vi "PwF_Venom_Open.vi"(8 "error in":errorcluster, 9 "Invert":bool, 10 "Device Number":u8) -> (0 "error out":errorcluster, 3 "Venom Ref":T1={"DeviceStatus"={"status"=FALSE, "code"=0, "source"=""}, "Type"=enum."PWM", "PWM"={"PWM Channel"=enum."PWM 1", "DeadBand"={"Name"="", "maxPositivePwm"=0, "minPositivePwm"=0, "centerPwm"=0, "maxNegativePwm"=0, "minNegativePwm"=0, "angularRange"=0}}, "CAN"={"Device Number"=0, "SetOutput VI Ref"=variant(enum8{"Percent VBus", "Current", "Speed", "Position", "Voltage"} enum."Percent VBus"), "GetOutput VI Ref"=variant(refnum<k1> refnum), "Enable VI Ref"=variant(dbl 12.0), "Disable VI Ref"=variant(enum8{"Percent VBus", "Speed", "Position", "Slave", "Unchanged / Invalid", "Voltage Compensation", "Current", "Motion Profile"} enum."Percent VBus"), "Data"=variant}, "Invert"=FALSE, "DIO PWM"={"PWM \"Enable\" Channel"=enum."Invalid", "DIOChannel"=enum."Invalid", "PWM Rate"=0.0}})   [LabVIEW 2018, in "PwF_Venom.lvlib"]
uses:
  PwF_Venom.lvlib
  <vilib>/Rock Robotics/WPI/MotorControl/WPI_MotorControlDeviceRef.ctl
  <vilib>/Rock Robotics/WPI/MotorControl/WPI_MotorControlType.ctl
  <vilib>/Rock Robotics/SystemInterfaces/DIO/FPGA_DIOPWMChannel.ctl
  <vilib>/Rock Robotics/WPI/PWM/WPI_PWMDeadband.ctl
  <vilib>/Rock Robotics/SystemInterfaces/DIO/FPGA_DIOChannel.ctl
  TypeDefs/PwF_Venom_DevRefData.ctl
  TypeDefs/PwF_Venom_ControlMode.ctl
  <vilib>/Rock Robotics/WPI/ThirdParty/Phoenix-LabVIEW/Controls/DriverLib.ctl
  <vilib>/Rock Robotics/SystemInterfaces/NetworkCommunication/NetComm_UsageReport_ResourceType.ctl
  PwF_Venom_WPISet.vi
  PwF_Venom_Disable.vi
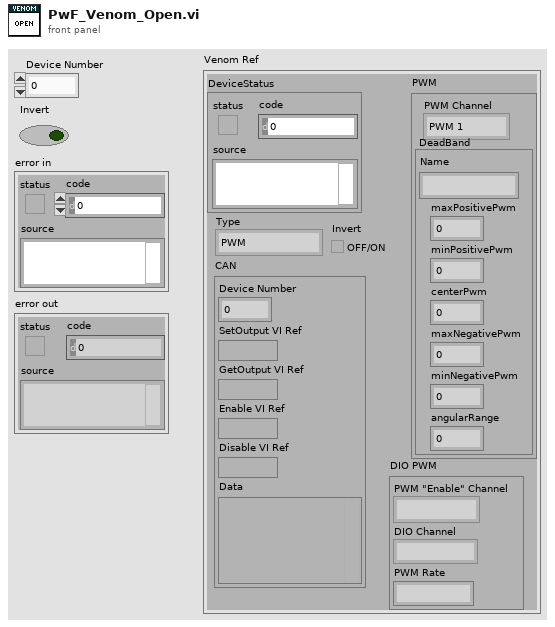
[diagram p1: front panel]
types:
  T1 = typedef "WPI_MotorControlDeviceRef.ctl" = cluster{"DeviceStatus":errorcluster, "Type":T2, "PWM":cluster{"PWM Channel":T3, "DeadBand":T4}, "CAN":cluster{"Device Number":u8, "SetOutput VI Ref":variant, "GetOutput VI Ref":variant, "Enable VI Ref":variant, "Disable VI Ref":variant, "Data":variant}, "Invert":bool, "DIO PWM":cluster{"PWM \"Enable\" Channel":T3, "DIOChannel":T5, "PWM Rate":dbl}}
  T2 = typedef "WPI_MotorControlType.ctl" = enum16{"PWM", "CAN", "DIO PWM"}
  T3 = typedef "FPGA_DIOPWMChannel.ctl" = enum8{"PWM 0", "PWM 1", "PWM 2", "PWM 3", "PWM 4", "PWM 5", "PWM 6", "PWM 7", "PWM 8", "PWM 9", "PWM MXP 0", "PWM MXP 1", "PWM MXP 2", "PWM MXP 3", "PWM MXP 4", "PWM MXP 5", "PWM MXP 6", "PWM MXP 7", "PWM MXP 8", "PWM MXP 9", "Invalid"}
  T4 = typedef "WPI_PWMDeadband.ctl" = cluster{"Name":string, "maxPositivePwm":i32, "minPositivePwm":i32, "centerPwm":i32, "maxNegativePwm":i32, "minNegativePwm":i32, "angularRange":u16}
  T5 = typedef "FPGA_DIOChannel.ctl" = enum8{"DIO 0", "DIO 1", "DIO 2", "DIO 3", "DIO 4", "DIO 5", "DIO 6", "DIO 7", "DIO 8", "DIO 9", "DIO MXP 0", "DIO MXP 1", "DIO MXP 2", "DIO MXP 3", "DIO MXP 4", "DIO MXP 5", "DIO MXP 6", "DIO MXP 7", "DIO MXP 8", "DIO MXP 9", "DIO MXP 10", "DIO MXP 11", "DIO MXP 12", "DIO MXP 13", "DIO MXP 14", "DIO MXP 15", "SPI Port CS1", "SPI Port CS2", "SPI Port CS3", "SPI Port MISO", "SPI Port MOSI", "Invalid"}
  T6 = typedef "PwF_Venom.lvlib/PwF_Venom_DevRefData.ctl" = cluster{"Library":path, "Handle":u64, "Control Mode":T7, "RefNum Name":string}
  T7 = typedef "PwF_Venom.lvlib/PwF_Venom_ControlMode.ctl" = u8
  T8 = typedef "NetComm_UsageReport_ResourceType.ctl" = enum8{"Controller", "Module", "Language", "CANPlugin", "Accelerometer", "ADXL345", "AnalogChannel", "AnalogTrigger", "AnalogTriggerOutput", "CANJaguar", "Compressor", "Counter", "Dashboard", "DigitalInput", "DigitalOutput", "DriverStationCIO", "DriverStationEIO", "DriverStationLCD", "Encoder", "GearTooth", "Gyro", "I2C", "Framework", "Jaguar", "Joystick", "Kinect", "KinectStick", "PIDController", "Preferences", "PWM", "Relay", "RobotDrive", "SerialPort", "Servo", "Solenoid", "SPI", "Task", "Ultrasonic", "Victor", "Button", "Command", "AxisCamera", "PCVideoServer", "SmartDashboard", "Talon", "HiTechnicColorSensor", "HiTechnicAccel", "HiTechnicCompass", "SRF08", "AnalogOutput", "Victor SP", "Talon SRX", "CAN Talon SRX", "ADXL362 Accel", "ADXRS450 Gyro", "Rev SPARK", "Mindsensors SD540", "Digital Filter", "ADIS16448", "PDP", "PCM", "PigeonIMU", "Nidec Brushless", "CTRE CANifier", "CTRE Future 0", "CTRE Future 1", "CTRE Future 2", "CTRE Future 3", "CTRE Future 4", "CTRE Future 5", "CTRE Future 6", "Linear Filter", "Xbox Controller", "USB Camera", "NavX", "Pixy", "Pixy2", "ScanseSweep", "Shuffleboard", "CAN", "Digilent DMC60", "PWM Victor SPX", "Rev SPARK MAX PWM", "Rev SPARK MAX CAN", "ADIS16470"}
  T9 = typedef "DriverLib.ctl" = path
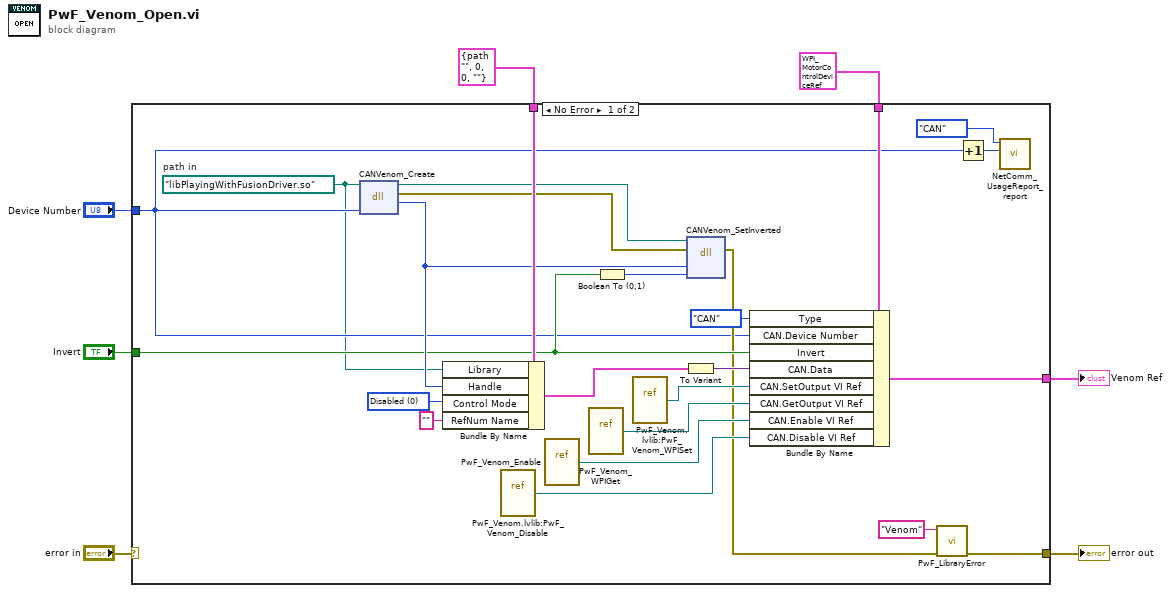
[diagram p0: block diagram]
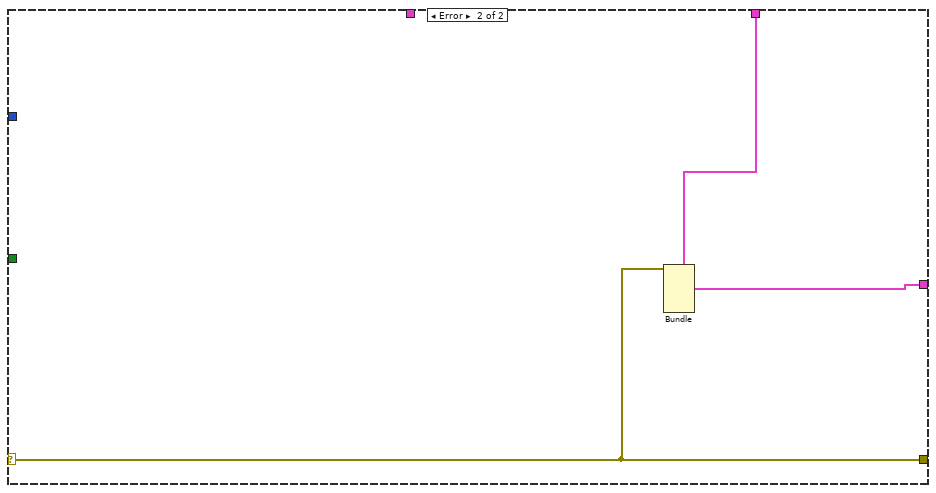
[diagram p2: hidden frame]
diagram:
  n1 = case shown="No Error" "error in" {
    selector: "error in" -> [_ w32]
    tunnel: [w17 w32] -> w7
    tunnel: "Invert" -> [w20 _]
    tunnel: T1 {"DeviceStatus"={"status"=FALSE, "code"=0, "source"=""}, "Type"=enum."CAN", "PWM"={"PWM Channel"=enum."PWM 1", "DeadBand"={"Name"="", "maxPositivePwm"=0, "minPositivePwm"=0, "centerPwm"=0, "maxNegativePwm"=0, "minNegativePwm"=0, "angularRange"=0}}, "CAN"={"Device Number"=0, "SetOutput VI Ref"=variant(refnum<vi> refnum), "GetOutput VI Ref"=variant(refnum<vi> refnum), "Enable VI Ref"=variant(refnum<vi> refnum), "Disable VI Ref"=variant(refnum<vi> refnum), "Data"=variant(cluster{"Control Mode":enum8{"Percent VBus", "Speed", "Position", "Slave", "Unchanged / Invalid", "Voltage Compensation", "Current", "Motion Profile"}, "Encoder Initial Position":dbl, "MaxVout":dbl} {"Control Mode"=enum."Percent VBus", "Encoder Initial Position"=0.0, "MaxVout"=12.0})}, "Invert"=FALSE, "DIO PWM"={"PWM \"Enable\" Channel"=enum."Invalid", "DIOChannel"=enum."Invalid", "PWM Rate"=0.0}} ("CAN Talon SRX Ref") -> [w31 w34]
    tunnel: "Device Number" -> [w12 _]
    tunnel: [w8 w33] -> w1
    tunnel: T6 {"Library"=path "", "Handle"=0, "Control Mode"=0, "RefNum Name"=""} -> [w23 _]
    frame No Error {
      w10 = T7 0 items=["Disabled"=0, "Proportional"=1, "Current Control"=3, "Speed Control"=4, "Position Control"=5, "Motion Profile"=6, "Follow The Leader"=7, "Voltage Control"=8] ("Control Mode")
      w9 = T9 path "libPlayingWithFusionDriver.so"  # path in
      n2 = dll-call lib="?" fn="CANVenom_Create"(path in=w9, "motorID"=w12) -> (path out=w13:path, error out=w16:errorcluster, "handle"=w21:u64)  [unwired: 3 in]
      n3 = Bundle By Name(cluster=w23, "Library"=w9, "Handle"=w21, "Control Mode"=w10, "RefNum Name"="") -> (w24:T6)
      n4 = vi-ref "PwF_Venom.lvlib:PwF_Venom_Disable.vi"() -> (w26:refnum<vi>)
      n5 = vi-ref "PwF_Venom_Enable.vi"() -> (w27:refnum<vi>)
      n6 = vi-ref "PwF_Venom_WPIGet.vi"() -> (w28:refnum<vi>)
      n7 = Boolean To (0,1)(Boolean=w20) -> (0, 1=w22:i16)
      n8 = vi-ref "PwF_Venom.lvlib:PwF_Venom_WPISet.vi"() -> (w29:refnum<vi>)
      n9 = To Variant(anything=w24) -> (Variant=w25:variant)
      n10 = dll-call lib="?" fn="CANVenom_SetInverted"(path in=w13, error in=w16, "handle"=w21, "isInverted"=w22) -> (error out=w19:errorcluster)  [unwired: 4 in, 1 out]
      n11 = Bundle By Name(cluster=w31, "Type"=WPI_MotorControlType."CAN", "CAN.Device Number"=w12, "Invert"=w20, "CAN.Data"=w25, "CAN.SetOutput VI Ref"=w29, "CAN.GetOutput VI Ref"=w28, "CAN.Enable VI Ref"=w27, "CAN.Disable VI Ref"=w26) -> (w8:T1)
      n12 = call "PwF_LibraryError.vi"("error in"=w19, "DeviceType"="Venom") -> ("error out"=w17:errorcluster)  [unwired: 9 in]
      n13 = Increment(x=w12) -> (x+1=w15:u8)
      n14 = call <vilib>:"NetComm_UsageReport_report.vi"("Instance Number"=w15, "Resource Type"=NetComm_UsageReport_ResourceType."CAN") -> ()  [unwired: 10 in]
    }
    frame Error {
      n15 = Bundle(cluster=w34, "DeviceStatus"=w32) -> (w33:T1)  [unwired: 5 in]
    }
  }
  "Venom Ref" <- w1
  "error out" <- w7
